vi "Create Evaluations.vi"(8 "error in (no error)":errorcluster, 11 "IEvaluation in":refnum<class "RxBN_CHP.lvclass">) -> (0 "error out":errorcluster, 2 "Evaluations Out":T1[](array[typedef]) {"Low Limit" format="%#_13g"; "SI Scaling" items=["femto"=-15, "pico"=-12, "nano"=-9, "micro"=-6, "milli"=-3, "percent"=-2, ""=0, "kilo"=3, "mega"=6, "giga"=9, "tera"=12]}, 3 "IEvaluation out":refnum<class "RxBN_CHP.lvclass">)   [LabVIEW 2016, in "SeqAuto Evaluations.lvlib" / "RxBN_CHP.lvclass"]
uses:
  RxBN_CHP.lvclass
  C:/projects/STS/Common/Sequence Automation/Plugins/SeqAuto IEvaluation.lvlibp/SeqAuto IEvaluation.lvclass
  Plugins/TestStand API Tools (TSAT).lvlibp/Evaluation Actions/Includes/Controls/TSAT Evaluation.ctl
  Plugins/TestStand API Tools (TSAT).lvlibp/Evaluation Actions/Includes/Controls/TSAT Eval SI Unit Scaling.ctl
  Plugins/TestStand API Tools (TSAT).lvlibp/Evaluation Actions/Includes/Controls/TSAT Evaluation Type.ctl
  RxBN_CHP.lvclass/RxBN_CHP.ctl
  Read SA Pin.vi
  Write Exported Data Location.vi
  Plugins/SeqAuto IEvaluation.lvlibp/Read Measurement Name.vi
  Plugins/TestStand API Tools (TSAT).lvlibp/Evaluation Actions/TSAT Evaluation Actions.lvlib
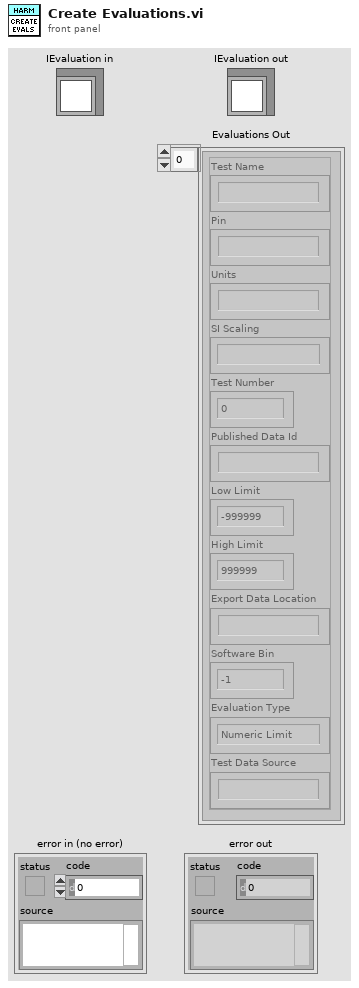
[diagram p1: front panel]
types:
  T1 = typedef "TestStand API Tools (TSAT).lvlibp/TSAT Evaluation Actions.lvlib/TSAT Evaluation.ctl" = cluster{"Test Name":string, "Pin":string, "Units":string, "SI Scaling":T2, "Test Number":i32, "Published Data Id":string, "Low Limit":dbl, "High Limit":dbl, "Export Data Location":string, "Software Bin":i64, "Evaluation Type":T3, "Test Data Source":string}
  T2 = typedef "TestStand API Tools (TSAT).lvlibp/TSAT Evaluation Actions.lvlib/TSAT Eval SI Unit Scaling.ctl" = i16
  T3 = typedef "TestStand API Tools (TSAT).lvlibp/TSAT Evaluation Actions.lvlib/TSAT Evaluation Type.ctl" = enum16{"Numeric Limit", "Pass/Fail", "None"}
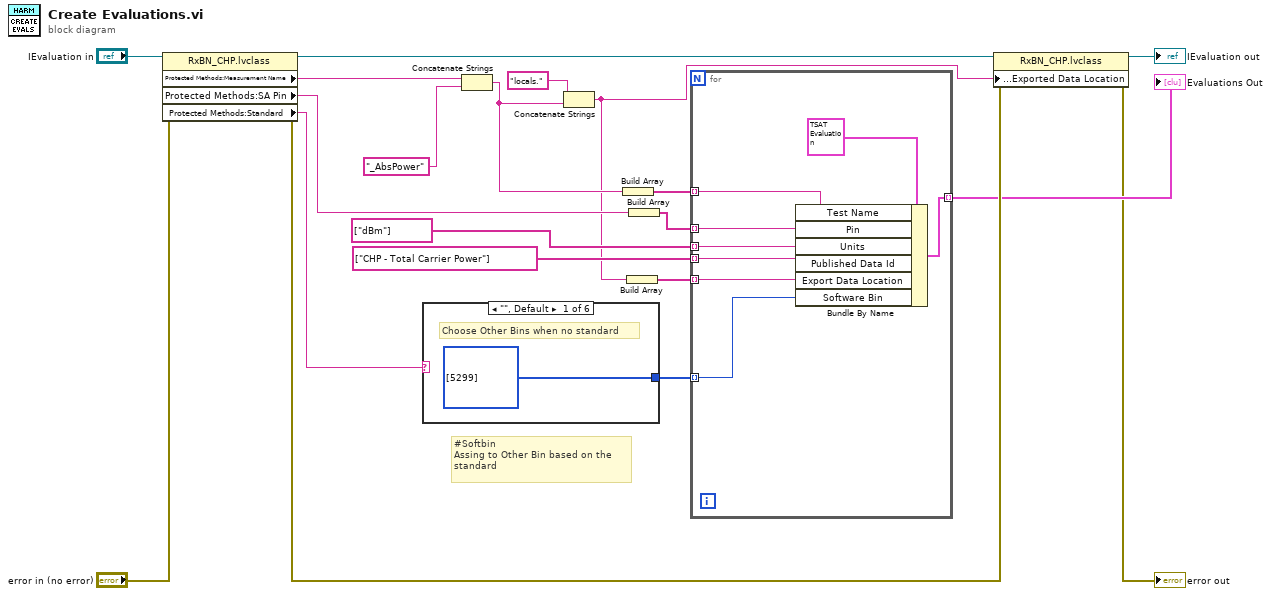
[diagram p0: block diagram]
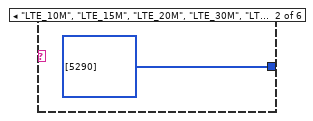
[diagram p2: hidden frame]
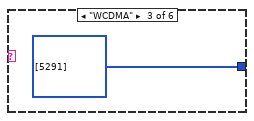
[diagram p3: hidden frame]
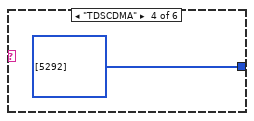
[diagram p4: hidden frame]
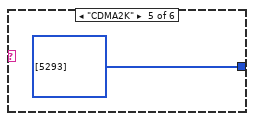
[diagram p5: hidden frame]
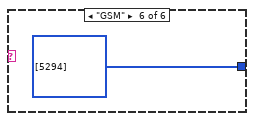
[diagram p6: hidden frame]
diagram:
  # "#Softbin\nAssing to Other Bin based on the \nstandard"
  n1 = property class="RxBN_CHP.lvclass"(reference="IEvaluation in", error in="error in (no error)") -> (reference out=w8:refnum<class "RxBN_CHP.lvclass">, error out=w19:errorcluster, "Protected Methods:Measurement Name"=w6:string, "Protected Methods:SA Pin"=w13:string, "Protected Methods:Standard"=w2:string)
  n2 = case shown="\"\", Default" w2 {
    tunnel: [i64[] [5299] i64[] [5290] i64[] [5291] i64[] [5292] i64[] [5293] i64[] [5294]] -> w1
    frame "", Default {
      # "Choose Other Bins when no standard"
    }
    frame "LTE_10M", "LTE_15M", "LTE_20M", "LTE_30M", "LTE_40M" {
    }
    frame "WCDMA" {
    }
    frame "TDSCDMA" {
    }
    frame "CDMA2K" {
    }
    frame "GSM" {
    }
  }
  n3 = Concatenate Strings(w6, "_AbsPower" ("string")) -> (w4:string)
  n4 = Concatenate Strings("locals." ("string"), w4) -> (w3:string)
  n5 = Build Array(w4) -> (w15:string[])
  n6 = Build Array(w3) -> (w14:string[])
  n7 = Build Array(w13) -> (w12:string[])
  n8 = for {
    tunnel: [w33] -> w17 mode=indexing
    tunnel: w15 -> [w32] mode=indexing
    tunnel: w14 -> [w31] mode=indexing
    tunnel: w12 -> [w30] mode=indexing
    tunnel: string[] ["dBm"] -> [w29] mode=indexing
    tunnel: string[] ["CHP - Total Carrier Power"] -> [w28] mode=indexing
    tunnel: w1 -> [w27] mode=indexing
    n9 = Bundle By Name(cluster=T1 {"Test Name"="", "Pin"="", "Units"="", "SI Scaling"=0, "Test Number"=0, "Published Data Id"="", "Low Limit"=-999999.0, "High Limit"=999999.0, "Export Data Location"="", "Software Bin"=-1, "Evaluation Type"=enum."Numeric Limit", "Test Data Source"=""} ("Evaluation"), "Test Name"=w32, "Pin"=w30, "Units"=w29, "Published Data Id"=w28, "Export Data Location"=w31, "Software Bin"=w27) -> (w33:T1)
  }
  "Evaluations Out" <- w17
  n10 = property class="RxBN_CHP.lvclass"(reference=w8, error in=w19, "Protected Methods:Exported Data Location"=w3) -> (reference out=→"IEvaluation out":refnum<class "RxBN_CHP.lvclass">, error out=→"error out":errorcluster)
